vi "STOP.vi"(8 "error in (no error)":errorcluster, 11 "Stop in":refnum<class "VIS-NIR_STRESING_NEW.lvclass">) -> (0 "error out":errorcluster, 3 "Stop out":refnum<class "VIS-NIR_STRESING_NEW.lvclass">)   [LabVIEW 2020, in "VIS-NIR_STRESING_NEW.lvclass"]
uses:
  VIS-NIR_STRESING_NEW/VIS-NIR_STRESING_NEW.lvclass
  C:/dev/TRANCON/Classes/GeneralFunctionality/GeneralFunctionality.lvclass
  GeneralFunctionality/GeneralFunctionality.lvclass/GeneralFunctionality.ctl
  GeneralFunctionality/GeneralFunctionality.lvclass
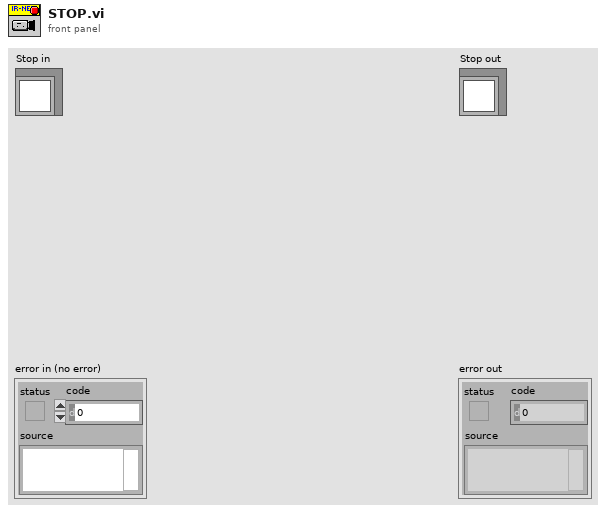
[diagram p1: front panel]
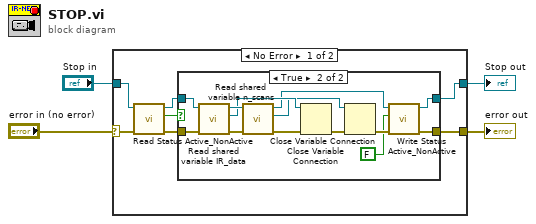
[diagram p0: block diagram]
diagram:
  n1 = case shown="No Error" "error in (no error)" {
    selector: "error in (no error)" -> [w9 w28]
    tunnel: [w10 w28] -> w2
    tunnel: "Stop in" -> [w8 w27]
    tunnel: [w11 w27] -> w3
    frame No Error {
      n2 = call "Read Status Active_NonActive.vi"("error in (no error)"=w9, "GeneralFunctionality in"=w8) -> ("error out"=w5:errorcluster, "Status Active/NonActive"=w7:bool, "GeneralFunctionality out"=w6:refnum<class "VIS-NIR_STRESING_NEW.lvclass">)  [unwired: 7 in]
      n3 = case shown="True" w7 {
        tunnel: [w13 w25] -> w11
        tunnel: [w12 w26] -> w10
        tunnel: w6 -> [w13 w18]
        tunnel: w5 -> [w12 w15]
        frame False {
        }
        frame True {
          n4 = call-dynamic "Read shared variable IR_data.vi"("error in (no error)"=w15, "VIS-NIR_STRESING_NEW in"=w18) -> ("error out"=w24:errorcluster, "shared variable IR_data"=w22:refnum<k21>, "VIS-NIR_STRESING_NEW out"=w23:refnum<class "VIS-NIR_STRESING_NEW.lvclass">)  [unwired: 7 in]
          n5 = call-dynamic "Read shared variable n_scans.vi"("error in (no error)"=w24, "VIS-NIR_STRESING_NEW in"=w23) -> ("error out"=w20:errorcluster, "shared variable n_scans"=w21:refnum<k21>, "VIS-NIR_STRESING_NEW out"=w17:refnum<class "VIS-NIR_STRESING_NEW.lvclass">)  [unwired: 7 in]
          n6 = Close Variable Connection(8:w20, 11:w22) -> (0:w19:errorcluster)
          n7 = Close Variable Connection(8:w19, 11:w21) -> (0:w16:errorcluster)
          n8 = call "Write Status Active_NonActive.vi"("error in (no error)"=w16, "Status Active/NonActive"=FALSE, "GeneralFunctionality in"=w17) -> ("error out"=w26:errorcluster, "GeneralFunctionality out"=w25:refnum<class "VIS-NIR_STRESING_NEW.lvclass">)  [unwired: 7 in]
        }
      }
    }
    frame Error {
    }
  }
  "error out" <- w2
  "Stop out" <- w3
